vi "Launcher.vi"() -> ()   [LabVIEW 2020]
uses:
  <userlib>/_NEVSTOP/Communicable State Machine(CSM)/_Support/GlobalEvent/GEvt-Convert Filter Rules - v1.0.vi
  <userlib>/_NEVSTOP/Communicable State Machine(CSM)/addons/INI-Static-Variable-Support/_Support/instances/_CSM - Read Log Filter Rules - v1.0.vi
  <userlib>/_NEVSTOP/Communicable State Machine(CSM)/_Support/GlobalEvent/LogFilter/SettingVIs/Set Global CSM Filter.vi
  <userlib>/_NEVSTOP/Communicable State Machine(CSM)/_Support/GlobalEvent/LogFilter/SettingVIs/Set Global LogType Filter.vi
  <userlib>/_NEVSTOP/Communicable State Machine(CSM)/_Support/GlobalEvent/LogFilter/SettingVIs/Set Global State Filter.vi
  <userlib>/_NEVSTOP/Communicable State Machine(CSM)/_Support/GlobalEvent/LogFilter/SettingVIs/Set CSM LogType Filter.vi
  <userlib>/_NEVSTOP/Communicable State Machine(CSM)/_Support/GlobalEvent/LogFilter/SettingVIs/Set CSM State Filter.vi
  <userlib>/_NEVSTOP/Communicable State Machine(CSM)/_Support/GlobalEvent/LogFilter/SettingVIs/Set Global StateType Filter.vi
  <userlib>/_NEVSTOP/Communicable State Machine(CSM)/_Support/GlobalEvent/LogFilter/SettingVIs/Set CSM StateType Filter.vi
  <userlib>/_NEVSTOP/Communicable State Machine(CSM)/addons/INI-Static-Variable-Support/_Support/instances/_CSM - Read File Logger Configuration - v1.0.vi
  resource/global-rc-strings.vi
  <userlib>/_NEVSTOP/Communicable State Machine(CSM)/_Support/GlobalEvent/LogFilter/LogFilter.lvclass
  <userlib>/_NEVSTOP/Communicable State Machine(CSM)/addons/Watchdog/CSM Watchdog.lvlib
  <userlib>/_NEVSTOP/Communicable State Machine(CSM)/addons/Logger/CSM File Logger.lvlib
  <userlib>/_NEVSTOP/Communicable State Machine(CSM)/Communicable State Machine.lvlib
  <userlib>/_NEVSTOP/Communicable State Machine(CSM)/addons/INI-Static-Variable-Support/INI-Static-Variable-Support.lvlib
  CSMScript-Engine(Lite).lvlib
panel:
  out "Information":string="Load \"csm\"..."
  out "CSMVersion":string="Powered By CSM, Copyright ?2025 NEVSTOP-LAB"
  out "CSMScript(version)":string="CSMScript-Lite"
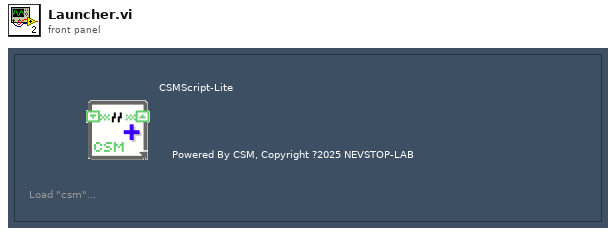
[diagram p1: front panel]
types:
  T1 = cluster{"Enable":bool, "Limit":cluster{"FileSize":i64, "FileNum":i32}, "Timestamp.Format":string, "AutoExit":bool}
  T2 = typedef "Communicable State Machine.lvlib/_CSM_GlobalLog Filter Rules - v1.0.ctl" = cluster{"Global":cluster{"CSM":string[], "LogType":T3[], "State":string[], "StateType":T4[]}, "CSM":cluster{"LogType":cluster{"CSM":string, "LogType":T3}[], "State":cluster{"CSM":string, "State":string}[], "StateType":cluster{"CSM":string, "LogType":T4}[]}}
  T3 = typedef "Communicable State Machine.lvlib/_CSM_GlobalLog_MSG_TYPE.ctl" = enum16{"User Log", "State Change", "Status", "Interrupt", "Register", "Unregister", "Error Log", "Module Created", "Module Destroyed", "Async Message", "No-Rep Async Message", "Sync Message", "AsyncMsg Complete", "SyncMsg Complete"}
  T4 = typedef "Communicable State Machine.lvlib/_CSM_GlobalLog_STATE_TYPE.ctl" = enum16{"State - Internal State", "State - External Message", "State - Response", "State - Complete"}
  T5 = enum32{"Invalid", "Standard", "Closed", "Hidden", "Minimized", "Maximized"}
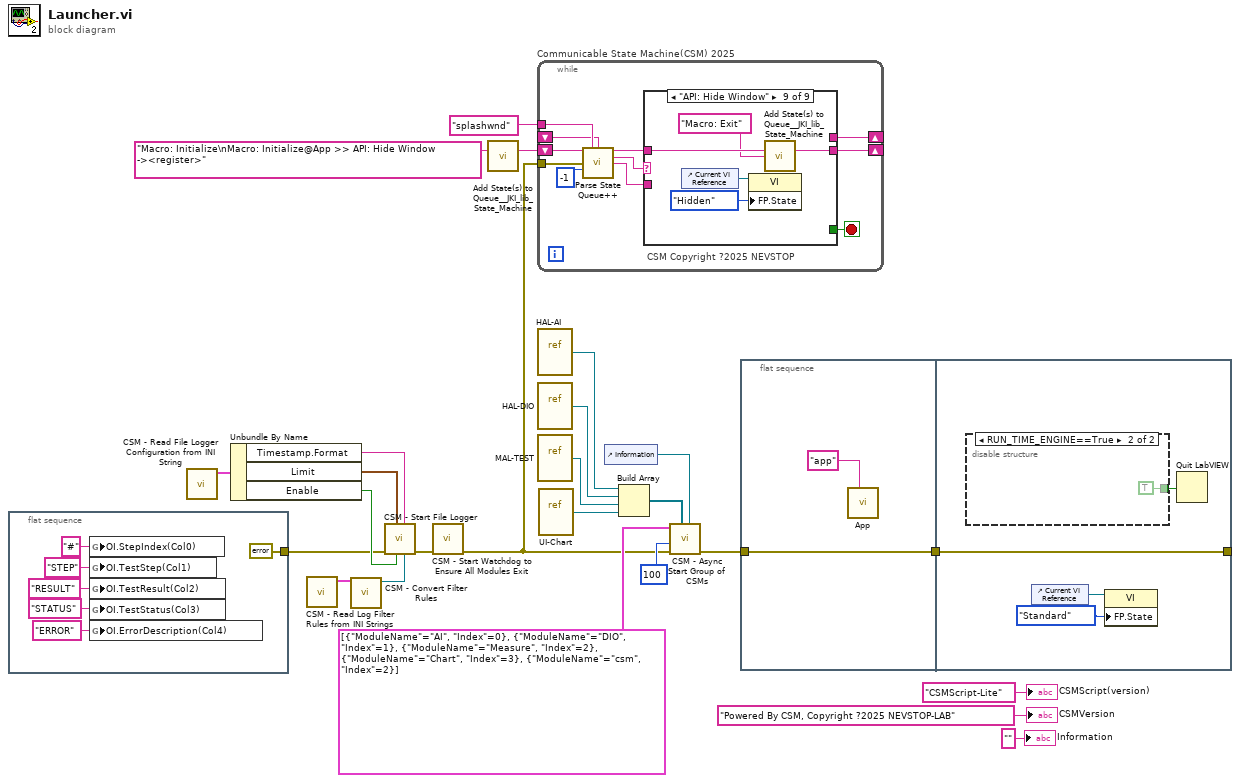
[diagram p0: block diagram]
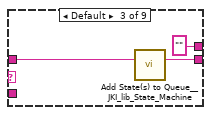
[diagram p4: hidden frame]
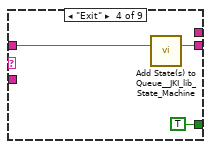
[diagram p5: hidden frame]
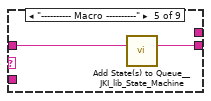
[diagram p6: hidden frame]
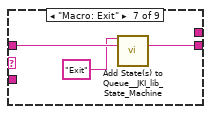
[diagram p8: hidden frame]
diagram:
  n1 = flat-sequence {
    tunnel: [errorcluster {"status"=FALSE, "code"=0, "source"=""} ("error in (no error)")] -> w5
    frame #0 {
      n2 = global write "global-rc-strings.vi" "OI.StepIndex(Col0)"("#" ("OI.StepIndex(Col0)")) -> ()
      n3 = global write "global-rc-strings.vi" "OI.TestStep(Col1)"("STEP" ("OI.TestStep(Col1)")) -> ()
      n4 = global write "global-rc-strings.vi" "OI.TestResult(Col2)"("RESULT" ("OI.TestResult(Col2)")) -> ()
      n5 = global write "global-rc-strings.vi" "OI.TestStatus(Col3)"("STATUS" ("OI.TestStatus(Col3)")) -> ()
      n6 = global write "global-rc-strings.vi" "OI.ErrorDescription(Col4)"("ERROR" ("OI.TestStatus(Col3)")) -> ()
    }
  }
  n7 = call-poly <userlib>:"CSM - Read File Logger Configuration from INI String.vi"() -> ("FileLogger Configuration-v1"=w15:T1)  [unwired: 8 in, 1 out]
  n8 = Unbundle By Name(w15) -> ("Timestamp.Format"=w12:string, "Limit"=w13:cluster{"FileSize":i64, "FileNum":i32}, "Enable"=w14:bool)
  n9 = call-poly <userlib>:"CSM - Read Log Filter Rules from INI Strings.vi"() -> ("Rules-v1"=w17:T2)  [unwired: 8 in, 1 out]
  n10 = call-poly <userlib>:"CSM - Convert Filter Rules.vi"("Rules-v1"=w17) -> ("GlobalLogFilter"=w18:refnum<class "LogFilter.lvclass">)  [unwired: 10 in]
  n11 = call <userlib>:"CSM - Start File Logger.vi"("Filter Rules"=w18, "Timestamp Format"=w12, "Enable? (T)"=w14, "Log Limit"=w13, "Error In"=w5) -> ("error out"=w11:errorcluster)  [unwired: 4 in, 2 out]
  n12 = call <userlib>:"CSM - Start Watchdog to Ensure All Modules Exit.vi"("error in (no error)"=w11) -> ("error out"=w1:errorcluster)  [unwired: 10 in]
  n13 = call <vilib>:"Add State(s) to Queue__JKI_lib_State_Machine.vi"("State(s) in (\"\")"="Macro: Initialize\nMacro: Initialize@App >> API: Hide Window -><register>" ("Init State(\"Macro: Initialize\")")) -> ("States Out"=w2:string)  [unwired: 14 in]
  n14 = while "Communicable State Machine(CSM) 2025" {
    shift-right: [w40] -> _
    shift-left: w2 -> [w41]
    tunnel: "splashwnd" ("Name (\"\" to Use UUID)") -> [w37]
    shift-right: [w38] -> _
    shift-left: _ -> [w34]
    tunnel: w1 -> [w32]
    stop <- w39 stop-if-true
    # "CSM Copyright ?2025 NEVSTOP"
    n15 = call <userlib>:"Parse State Queue++.vi"("State Queue"=w41, "Name (\"\" to Use UUID)"=w37, "Response Arguments"=w34, "Previous Error"=w32, "Dequeue (1 ms)"=-1 ("Timeout")) -> ("Remaining States"=w42:string, "Current State"=w36:string, "Arguments"=w35:string)  [unwired: 5 in, 3 out]
    n16 = case shown="\"API: Hide Window\"" w36 {
      tunnel: w42 -> [w43 w44 w47 w50 w52 w53 w56 w57 w59]
      tunnel: w35 -> [_ _ _ _ _ _ _ _ _]
      tunnel: [w43 w44 w46 w49 w51 w53 w55 w57 w60] -> w40
      tunnel: [_ _ _ TRUE _ _ _ _ _] -> w39
      tunnel: [_ _ "" _ _ _ _ _ _] -> w38
      frame "", "Idle" {
      }
      frame "---------- Core ----------" {
      }
      frame Default {
        n17 = call <vilib>:"Add State(s) to Queue__JKI_lib_State_Machine.vi"("State(s) in (\"\")"=w47) -> ("States Out"=w46:string)  [unwired: 14 in]
      }
      frame "Exit" {
        n18 = call <vilib>:"Add State(s) to Queue__JKI_lib_State_Machine.vi"("State(s) in (\"\")"=w50) -> ("States Out"=w49:string)  [unwired: 14 in]
      }
      frame "---------- Macro ----------" {
        n19 = call <vilib>:"Add State(s) to Queue__JKI_lib_State_Machine.vi"("State(s) in (\"\")"=w52) -> ("States Out"=w51:string)  [unwired: 14 in]
      }
      frame "Macro: Initialize" {
      }
      frame "Macro: Exit" {
        n20 = call <vilib>:"Add State(s) to Queue__JKI_lib_State_Machine.vi"("State(s) in Front (\"\")"="Exit", "State(s) in (\"\")"=w56) -> ("States Out"=w55:string)  [unwired: 13 in]
      }
      frame "---------- API ----------" {
      }
      frame "API: Hide Window" {
        n21 = control-ref of="Current VI Reference"() -> (w61:refnum<vi>)
        n22 = property class="VI"(reference=w61, "FP.State"=T5."Hidden" ("Front Panel Window:State")) -> ()  [unwired: 1 in, 2 out]
        n23 = call <vilib>:"Add State(s) to Queue__JKI_lib_State_Machine.vi"("State(s) in (\"\")"=w59, "State(s) at Back (\"\")"="Macro: Exit" ("State(s) in Front (\"\")")) -> ("States Out"=w60:string)  [unwired: 13 in]
      }
    }
  }
  n24 = vi-ref "HAL-AI.vi"() -> (w25:refnum<vi>)
  n25 = vi-ref "HAL-DIO.vi"() -> (w24:refnum<vi>)
  n26 = vi-ref "MAL-TEST.vi"() -> (w23:refnum<vi>)
  n27 = vi-ref "UI-Chart.vi"() -> (w19:refnum<vi>)
  n28 = control-ref of="Information"() -> (w7:refnum<vi>)
  n29 = Build Array(w25, w24, w23, w19) -> (w9:refnum<vi>[])
  n30 = call "CSM - Async Start Group of CSMs.vi"("Information"=w7, "Prototypes"=w9, "error in (no error)"=w1, "interval(50ms)"=u32 100, "Module List"=cluster{"ModuleName":string, "Index":i32}[] [{"ModuleName"="AI", "Index"=0}, {"ModuleName"="DIO", "Index"=1}, {"ModuleName"="Measure", "Index"=2}, {"ModuleName"="Chart", "Index"=3}, {"ModuleName"="csm", "Index"=2}]) -> ("error out"=w22:errorcluster)  [unwired: 4 in]
  n31 = flat-sequence {
    tunnel: [w64] -> w16
    tunnel: w22 -> [w64]
    tunnel: [w68] -> _
    tunnel: w16 -> [w68]
    frame #0 {
      n32 = call "App.vi"("Name(\"\" to use uuid)"="app" ("Name(\"\" to use uuid)")) -> ()  [unwired: 11 in]
    }
    frame #1 {
      n33 = disable-structure shown="RUN_TIME_ENGINE==True" {
        disable-tunnel: [_ TRUE ("quit? (T)")] -> w67
        frame condition #0 (active) {
        }
        frame condition #1 {
        }
      }
      n34 = control-ref of="Current VI Reference"() -> (w65:refnum<vi>)
      n35 = property class="VI"(reference=w65, "FP.State"=T5."Standard" ("Front Panel Window:State")) -> ()  [unwired: 1 in, 2 out]
      n36 = Quit LabVIEW(quit? (T)=w67) -> ()
    }
  }
  "CSMScript(version)" <- "CSMScript-Lite" ("String to Prepend to Source (\"\")")
  "CSMVersion" <- "Powered By CSM, Copyright ?2025 NEVSTOP-LAB" ("String to Prepend to Source (\"\")")
  "Information" <- "" ("Information")
